vi "WritePortStatus.vi"(8 "error in (no error)":errorcluster, 9 "Value":string, 10 "Port":dbl, 11 "NXP in":refnum<class "NXP.lvclass">) -> (0 "error out":errorcluster, 3 "NXP out":refnum<class "NXP.lvclass">)   [LabVIEW 2020, in "NXP.lvclass"]
uses:
  NXP.lvclass
  Abstract/Serial Device/Serial Device.lvclass
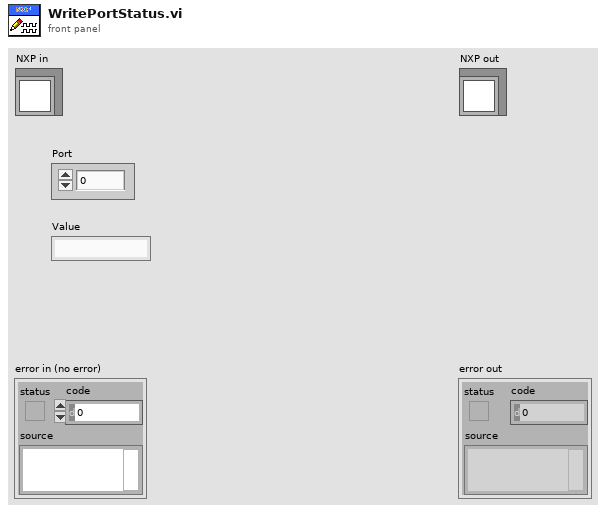
[diagram p1: front panel]
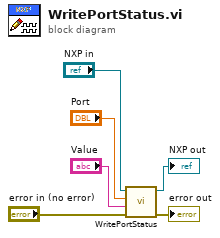
[diagram p0: block diagram]
diagram:
  n1 = call-parent "WritePortStatus.vi"("error in (no error)"="error in (no error)", "Value"="Value", "Port"="Port", "Serial Device in"="NXP in") -> ("error out"=→"error out":errorcluster, "Serial Device out"=→"NXP out":refnum<class "NXP.lvclass">)  [unwired: 6 in]
